vi "Set Panel BG.vi"(8 "error in (no error)":errorcluster, 10 "Pane Color":u32(colorbox), 11 "[V] Main UI in":refnum<class "[V] Main UI.lvclass">) -> (0 "error out":errorcluster, 3 "[V] Main UI out":refnum<class "[V] Main UI.lvclass">)   [LabVIEW 2020, in "[V] Main UI.lvlib" / "[V] Main UI.lvclass"]
uses:
  [V] Main UI.lvclass
  Depden On/Abstruct View/Abstruct View/Abstruct View.lvclass/Abstruct View.ctl
  Depden On/Abstruct View/Abstruct View/Data Accessors/Read Core VI.vi
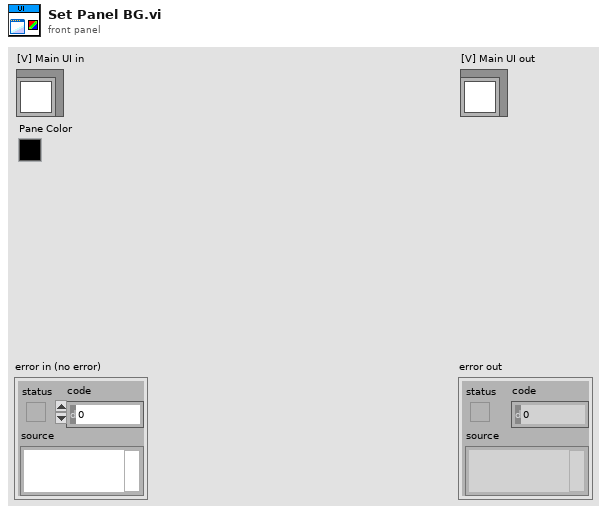
[diagram p1: front panel]
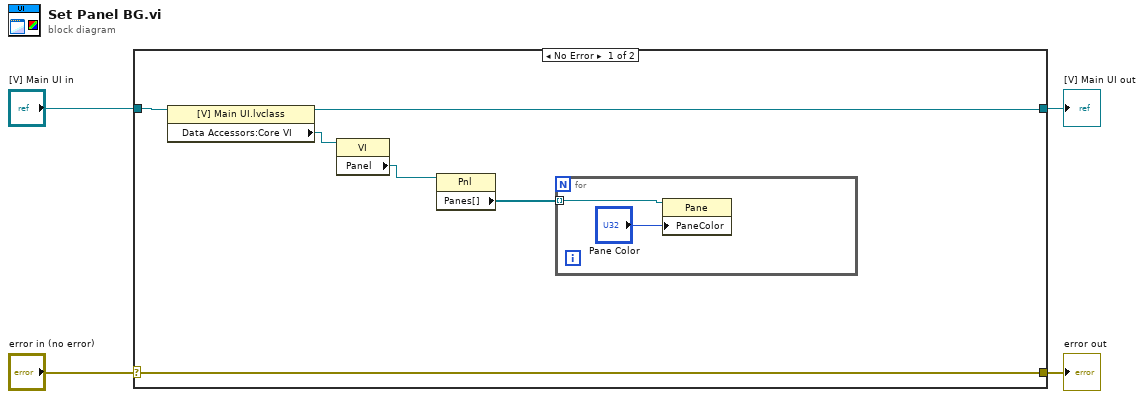
[diagram p0: block diagram]
diagram:
  n1 = case shown="No Error" "error in (no error)" {
    selector: "error in (no error)" -> [w10 w14]
    tunnel: [w10 w14] -> w3
    tunnel: [w8 w13] -> w1
    tunnel: "[V] Main UI in" -> [w9 w13]
    frame No Error {
      n2 = property class="[V] Main UI.lvclass"(reference=w9) -> (reference out=w8:refnum<class "[V] Main UI.lvclass">, "Data Accessors:Core VI"=w7:refnum<vi>)  [unwired: 1 in, 1 out]
      n3 = property class="VI"(reference=w7) -> ("Panel"=w5:refnum<vi>)  [unwired: 1 in, 2 out]
      n4 = property class="Pnl"(reference=w5) -> ("Panes[]"=w6:refnum<vi>[])  [unwired: 1 in, 2 out]
      n5 = for {
        tunnel: w6 -> [w12] mode=indexing
        n6 = property class="Pane"(reference=w12, "PaneColor"="Pane Color") -> ()  [unwired: 1 in, 2 out]
      }
    }
    frame Error {
    }
  }
  "error out" <- w3
  "[V] Main UI out" <- w1
